vi "PresaAvandaroAnalogica.vi"() -> ()   [LabVIEW 2018]
uses:
  EdoPresaAnalogica.ctl
panel:
  out "Edo":T1
  in  "stop":bool
  out "Motor2":dbl(knob) scale=0.0..10.0
  out "Motor1":dbl(knob) scale=0.0..10.0
  in  "Presa":dbl(slide) scale=0.0..100.0
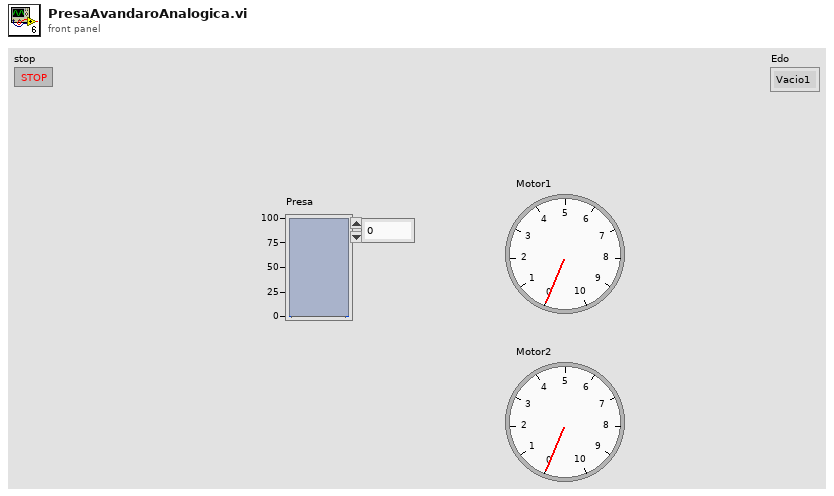
[diagram p1: front panel]
types:
  T1 = typedef "EdoPresaAnalogica.ctl" = enum16{"Vacio1", "Mitad1", "Vacio2", "Mitad2", "Lleno1", "Lleno2"}
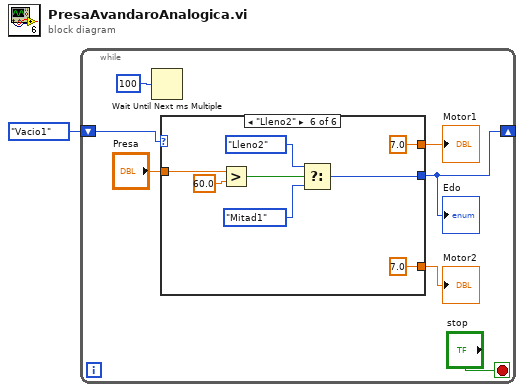
[diagram p0: block diagram]
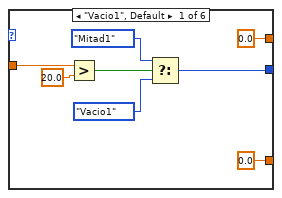
[diagram p2: hidden frame]
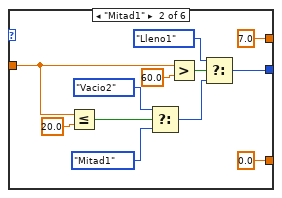
[diagram p3: hidden frame]
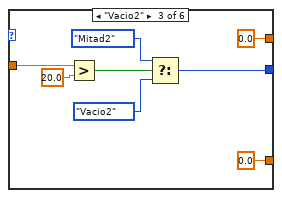
[diagram p4: hidden frame]
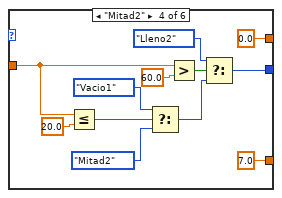
[diagram p5: hidden frame]
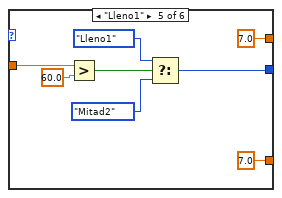
[diagram p6: hidden frame]
diagram:
  n1 = while {
    shift-right: [w4] -> _
    shift-left: EdoPresaAnalogica."Vacio1" -> [w6]
    stop <- "stop" stop-if-true
    n2 = Wait Until Next ms Multiple(millisecond multiple=u32 100) -> ()  [unwired: 1 out]
    n3 = case shown="\"Lleno2\"" w6 {
      tunnel: "Presa" -> [w16 w23 w36 w44 w54 w62]
      tunnel: [w11 w19 w31 w39 w49 w57] -> w4
      tunnel: [0.0 7.0 0.0 0.0 7.0 7.0] -> w3
      tunnel: [0.0 0.0 0.0 7.0 7.0 7.0] -> w2
      frame "Vacio1", Default {
        n4 = Greater?(x=w16, y=20.0) -> (0:w14:bool)
        n5 = Select(t=EdoPresaAnalogica."Mitad1", s=w14, f=EdoPresaAnalogica."Vacio1") -> (s? t:f=w11:T1)
      }
      frame "Mitad1" {
        n6 = Less Or Equal?(x=w23, y=20.0) -> (x <= y?=w24:bool)
        n7 = Select(t=EdoPresaAnalogica."Vacio2", s=w24, f=EdoPresaAnalogica."Mitad1") -> (s? t:f=w28:T1)
        n8 = Greater?(x=w23, y=60.0) -> (0:w26:bool)
        n9 = Select(t=EdoPresaAnalogica."Lleno1", s=w26, f=w28) -> (s? t:f=w19:T1)
      }
      frame "Vacio2" {
        n10 = Greater?(x=w36, y=20.0) -> (0:w34:bool)
        n11 = Select(t=EdoPresaAnalogica."Mitad2", s=w34, f=EdoPresaAnalogica."Vacio2") -> (s? t:f=w31:T1)
      }
      frame "Mitad2" {
        n12 = Less Or Equal?(x=w44, y=20.0) -> (x <= y?=w42:bool)
        n13 = Select(t=EdoPresaAnalogica."Vacio1", s=w42, f=EdoPresaAnalogica."Mitad2") -> (s? t:f=w48:T1)
        n14 = Greater?(x=w44, y=60.0) -> (0:w46:bool)
        n15 = Select(t=EdoPresaAnalogica."Lleno2", s=w46, f=w48) -> (s? t:f=w39:T1)
      }
      frame "Lleno1" {
        n16 = Greater?(x=w54, y=60.0) -> (0:w52:bool)
        n17 = Select(t=EdoPresaAnalogica."Lleno1", s=w52, f=EdoPresaAnalogica."Mitad2") -> (s? t:f=w49:T1)
      }
      frame "Lleno2" {
        n18 = Greater?(x=w62, y=60.0) -> (0:w60:bool)
        n19 = Select(t=EdoPresaAnalogica."Lleno2", s=w60, f=EdoPresaAnalogica."Mitad1") -> (s? t:f=w57:T1)
      }
    }
    "Motor1" <- w3
    "Motor2" <- w2
    "Edo" <- w4
  }
